vi "SubVI_SVM_Features_no_Maha.vi"(9 "dt":dbl=0.05 format="%#_13g", 10 "window_time":dbl[](array[numeric]), 11 "Sliding_window":dbl[](array[numeric])) -> (1 "min value":dbl, 2 "Features_array":dbl[](array[numeric]), 3 "slope":dbl, 4 "Trap Integrate":dbl format="%0.4f")   [LabVIEW 2020]
uses:
  <vilib>/Analysis/2dsp.llb/Integral Method.ctl
  <vilib>/Analysis/8numeric.llb/1D Numeric Integration.vi
  <vilib>/Analysis/NI_AALPro.lvlib
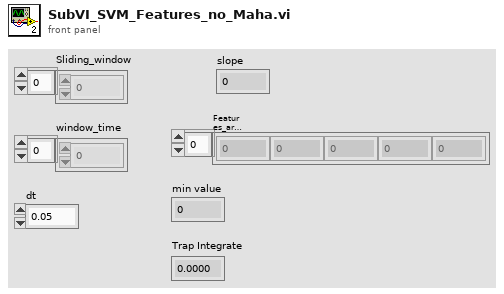
[diagram p1: front panel]
types:
  T1 = typedef "NI_AALPro.lvlib/Integral Method.ctl" = i32
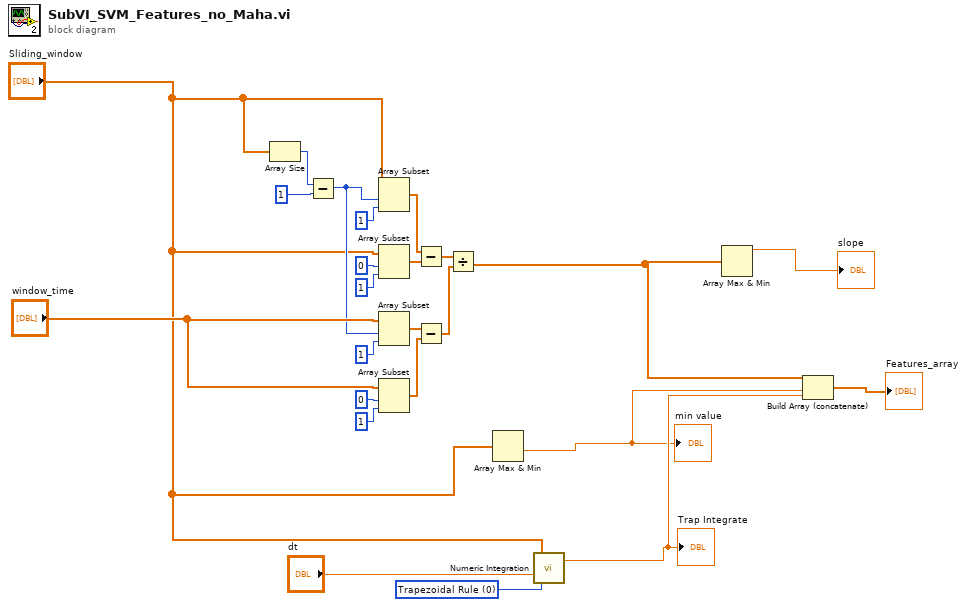
[diagram p0: block diagram]
diagram:
  w20 = T1 0 items=["Trapezoidal Rule", "Simpson's Rule", "Simpson's 3/8 Rule", "Bode Rule"] ("integration method")
  n1 = Array Size(array="Sliding_window") -> (size(s)=w6:i32)
  n2 = Subtract(x=w6, y=1 ("length")) -> (x-y=w4:i32)
  n3 = Array Subset(array="Sliding_window", index=w4, length=1) -> (w10:dbl[])
  n4 = Array Subset(array="Sliding_window", index=0, length=1) -> (w11:dbl[])
  n5 = Array Subset(array="window_time", index=w4, length=1) -> (w15:dbl[])
  n6 = Array Subset(array="window_time", index=0, length=1) -> (w16:dbl[])
  n7 = Subtract(x=w10, y=w11) -> (x-y=w17:dbl[])
  n8 = Subtract(x=w15, y=w16) -> (x-y=w18:dbl[])
  n9 = Divide(x=w17, y=w18) -> (x/y=w3:dbl[])
  n10 = Array Max & Min(array="Sliding_window") -> (min value=w21:dbl)  [unwired: 3 out]
  "min value" <- w21
  n11 = call-poly <vilib>:"Numeric Integration.vi"("integration method"=w20, "dt"="dt", "Input Array"="Sliding_window") -> ("result"=w22:dbl)  [unwired: 1 out]
  "Trap Integrate" <- w22
  n12 = Array Max & Min(array=w3) -> (max value=→"slope":dbl)  [unwired: 3 out]
  n13 = Build Array (concatenate)(w3, w21, w22) -> (→"Features_array":dbl[])
